vi "Error Query.vi"(8 "error in (no error)":errorcluster, 11 "VISA resource name":refnum<visa-resource-name>) -> (0 "error out":errorcluster, 1 "Error Code":i32, 2 "Error Message":string, 3 "VISA resource name out":refnum<visa-resource-name>)   [LabVIEW 2010, in "VITREK V7X.lvlib"]
doc: "Queries the instrument for any errors in the instrument's error queue. It will continue to read errors until all errors have been read from the instrument. Any errors will be returned in the <B>error out</B> control.\n\nNote:\nThis VI is called automatically by most driver VIs so it is not usually necessary to call this in an application."
uses:
  VITREK V7X.lvlib
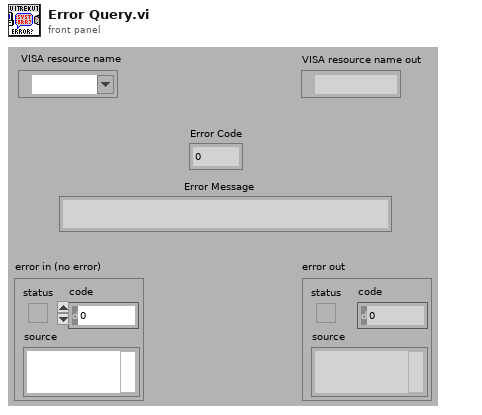
[diagram p1: front panel]
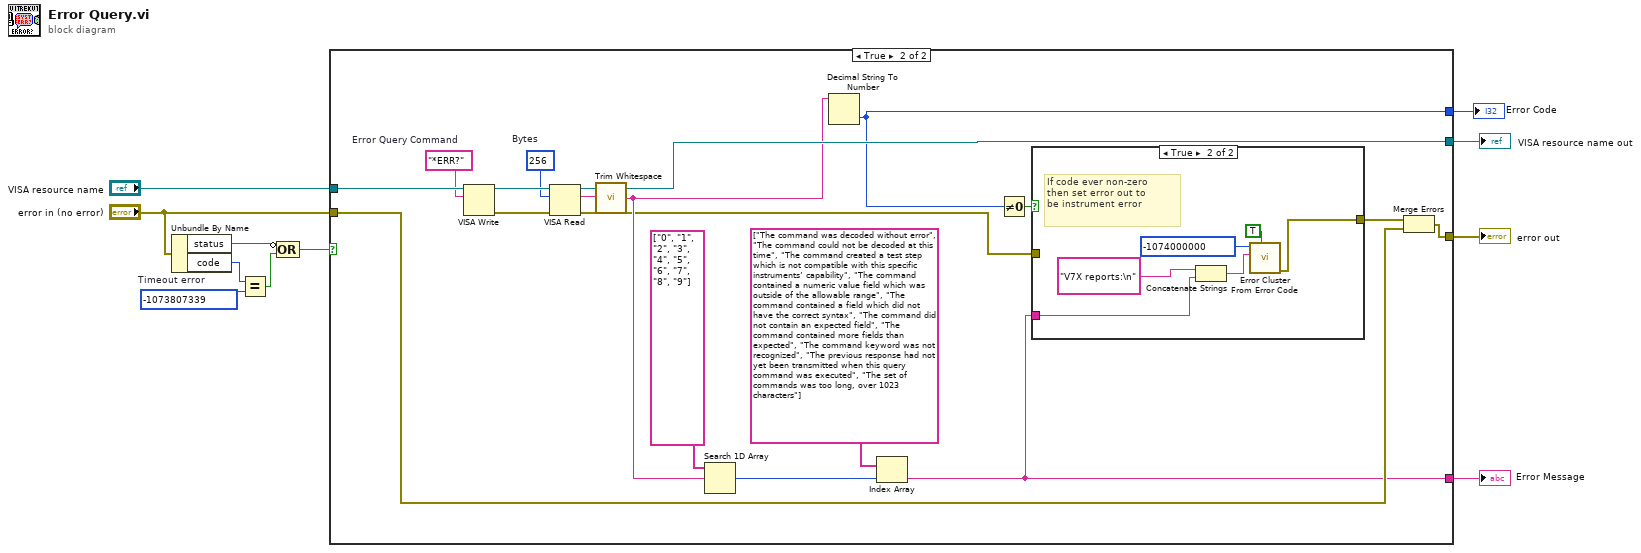
[diagram p0: block diagram]
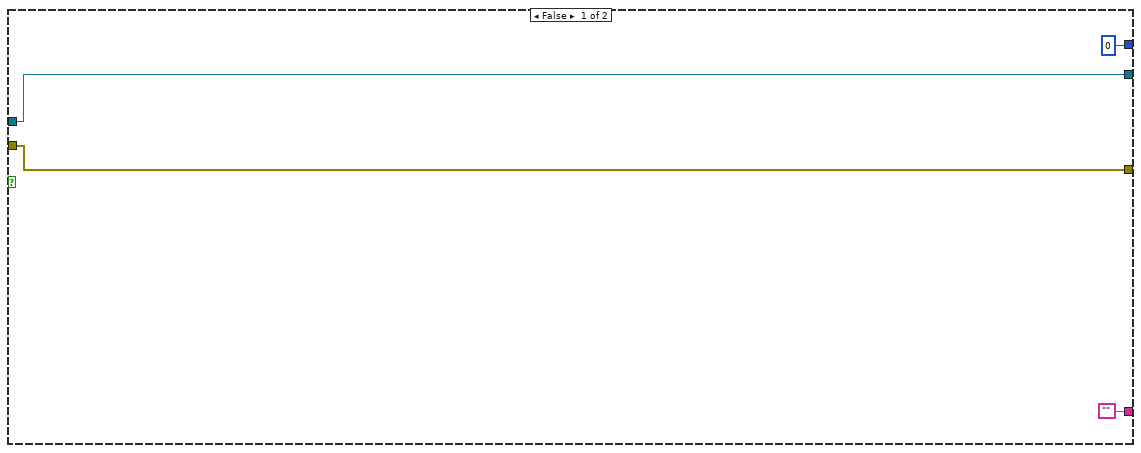
[diagram p2: hidden frame]
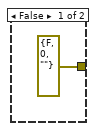
[diagram p3: hidden frame]
diagram:
  w6 = -1073807339  # Timeout error
  n1 = Unbundle By Name("error in (no error)") -> ("status"=w7:bool, "code"=w4:i32)
  n2 = Equal?(x=w4, y=w6) -> (x = y?=w5:bool)
  n3 = Compound Arithmetic op=OR(invert w7, w5) -> (w3:bool)
  n4 = case shown="True" w3 {
    tunnel: [w15 w33] -> w11
    tunnel: "VISA resource name" -> [w15 w32]
    tunnel: "error in (no error)" -> [w14 w28]
    tunnel: [w14 w31] -> w9
    tunnel: ["" w17] -> w2
    tunnel: [0 w16] -> w1
    frame False {
    }
    frame True {
      w26 = u32 256  # Bytes
      w24 = "*ERR?"  # Error Query Command
      n5 = VISA Write(VISA resource name=w32, write buffer=w24) -> (VISA resource name out=w27:refnum<visa-resource-name>, error out=w25:errorcluster)  [unwired: 1 in, 1 out]
      n6 = VISA Read(VISA resource name=w27, byte count=w26, error in (no error)=w25) -> (VISA resource name out=w33:refnum<visa-resource-name>, read buffer=w20:string, error out=w18:errorcluster)  [unwired: 1 out]
      n7 = call <vilib>:"Trim Whitespace.vi"("string"=w20) -> ("trimmed string"=w19:string)  [unwired: 1 in]
      n8 = Search 1D Array(1D array=string[] ["0", "1", "2", "3", "4", "5", "6", "7", "8", "9"], element=w19) -> (index of element=w21:i32)  [unwired: 1 in]
      n9 = Decimal String To Number(string=w19) -> (number=w16:i32)  [unwired: 2 in, 1 out]
      n10 = Index Array(array=string[] ["The command was decoded without error", "The command could not be decoded at this time", "The command created a test step which is not compatible with this specific instruments’ capability", "The command contained a numeric value field which was outside of the allowable range", "The command contained a field which did not have the correct syntax", "The command did not contain an expected field", "The command contained more fields than expected", "The command keyword was not recognized", "The previous response had not yet been transmitted when this query command was executed", "The set of commands was too long, over 1023 characters"], index=w21) -> (element=w17:string)
      n11 = Not Equal To 0?(x=w16) -> (x != 0?=w30:bool)
      n12 = case shown="True" w30 {
        tunnel: w17 -> [_ w39]
        tunnel: [errorcluster {"status"=FALSE, "code"=0, "source"=""} ("error out") w35] -> w29
        tunnel: w18 -> [_ _]
        frame False {
        }
        frame True {
          # "If code ever non-zero\nthen set error out to\nbe instrument error"
          n13 = Concatenate Strings("V7X reports:\n" ("Source"), w39) -> (w36:string)
          n14 = call <vilib>:"Error Cluster From Error Code.vi"("show call chain? (False)"=TRUE, "error message (\"\")"=w36, "error code (0)"=-1074000000 ("Code")) -> ("error out"=w35:errorcluster)  [unwired: 6 in]
        }
      }
      n15 = Merge Errors(w29, w28) -> (w31:errorcluster)
    }
  }
  "VISA resource name out" <- w11
  "error out" <- w9
  "Error Message" <- w2
  "Error Code" <- w1
